vi "LKIF2_GetSamplingRate.vi"(8 "error in":errorcluster) -> (0 "error out":errorcluster, 3 "Sampling Rate":T1)   [LabVIEW 2013, in "Keyence LK-G5000.lvlib"]
uses:
  <instrlib>/Keyence LK-G5000/Keyence LK-G5000.lvlib
  <instrlib>/Keyence LK-G5000/Public/enum/LKIF_SamplingRate.ctl
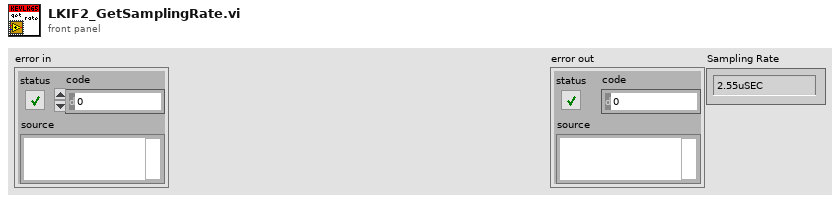
[diagram p1: front panel]
types:
  T1 = typedef "Keyence LK-G5000.lvlib/LKIF_SamplingRate.ctl" = enum16{"2.55uSEC", "5uSEC", "10uSEC", "20uSEC", "50uSEC", "100uSEC", "200uSEC", "500uSEC", "1mSEC"}
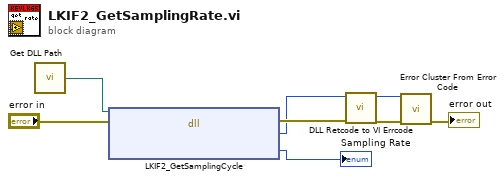
[diagram p0: block diagram]
diagram:
  n1 = call <instrlib>:"Get DLL Path.vi"() -> ("DLL Path"=w6:path)  [unwired: 1 in]
  n2 = dll-call lib="C:/Program Files (x86)/National Instruments/LabVIEW 2013/instr.lib/Keyence LK-G5000/LKIF2.dll" fn="LKIF2_GetSamplingCycle"(path in=w6, error in="error in") -> (error out=w5:errorcluster, "RC"=w4:i32, "SamplingCycle"=→"Sampling Rate":u16)  [unwired: 2 in, 1 out]
  n3 = call <instrlib>:"DLL Retcode to VI Errcode.vi"("error in (no error)"=w5, "DLL Retcode"=w4) -> ("error out"=w7:errorcluster, "VI Errcode"=w8:i32)  [unwired: 8 in]
  n4 = call <vilib>:"Error Cluster From Error Code.vi"("error in (no error)"=w7, "error code (0)"=w8) -> ("error out"=→"error out":errorcluster)  [unwired: 7 in]
